vi "demoYouTubeCDSim.vi"() -> ()   [LabVIEW 2020]
uses:
  <vilib>/addons/Control Design/_Model Construction/Model Creation.llb/Model Creation SubVI/cd_Create Transfer Function Model.vi
  <vilib>/addons/Control Design/_Utility/Model Viewer.llb/Model Viewer SubVI/cd_Draw Transfer Function Equation (TF).vi
  <vilib>/addons/Control Design/_Model Construction/NI_LinSys_Model Creation.lvlib
  <vilib>/addons/Control Design/_Utility/NI_CD_Model Viewer.lvlib
panel:
  in  "Delay (custom)":dbl format="%#_13g"
  in  "Denominator Coeffs (custom)":dbl[](array[numeric])=[1.0, 4.0, 8.0, 7.0]
  in  "Numerator Coeffs (custom)":dbl[](array[numeric])=[10.0, 5.0]
  out "Transfer Function Eqn":picture
  in  "Which Transfer Function Do You Want?":T1(ring)
  in  "Stop Program":bool
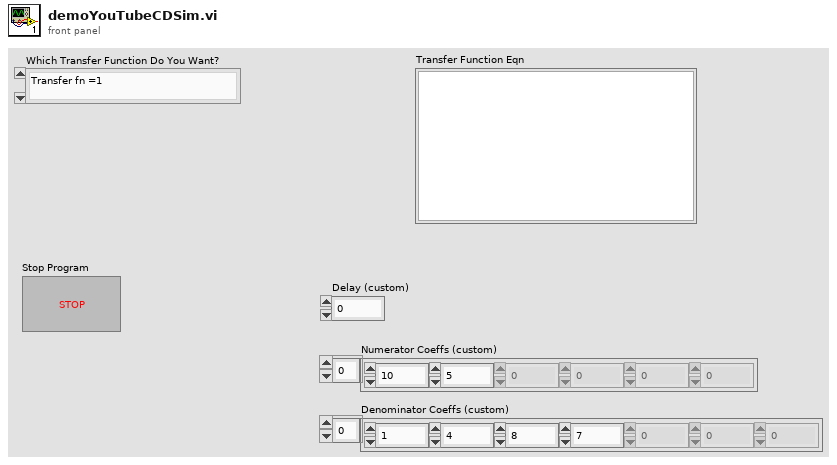
[diagram p1: front panel]
types:
  T1 = enum16{"Transfer fn =1", "first order with delay", "second order", "third order", "custom 1", "test 1", "test 2", "test 3", "test 4", "test 5", "test 6", "test 7", "test 8", "test 9", "test 10", ""}
  T2 = typedef "NI_LinSys_Model Typedefs.lvlib/CD Transfer Function Model (MIMO).ctl" = cluster{"properties":T3, "transfer function(s)":T4[][]}
  T3 = typedef "NI_LinSys_Model Typedefs.lvlib/CD General Elements.ctl" = cluster{"Model name":string, "Input names":string[], "Output names":string[], "Input Delays":dbl[], "Output Delays":dbl[], "Sampling Time":dbl, "Notes":string}
  T4 = typedef "NI_LinSys_Model Typedefs.lvlib/CD Transfer Function Model (SISO).ctl" = cluster{"Numerator":dbl[], "Denominator":dbl[], "delay":dbl}
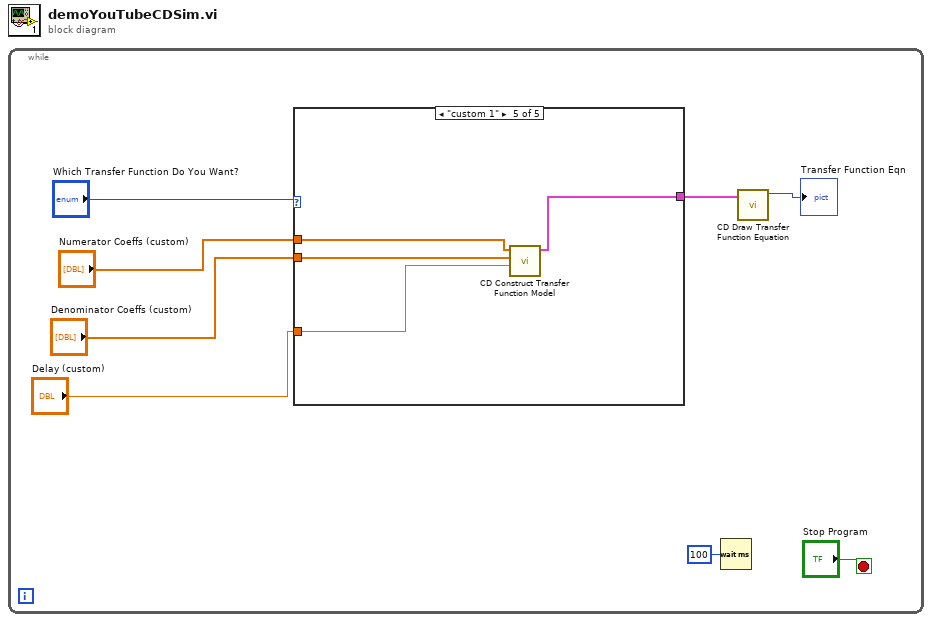
[diagram p0: block diagram]
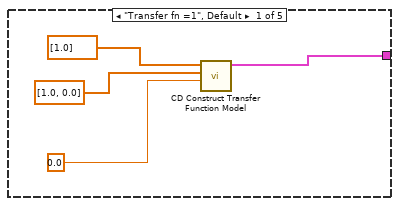
[diagram p2: hidden frame]
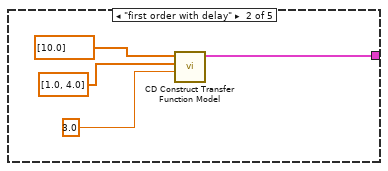
[diagram p3: hidden frame]
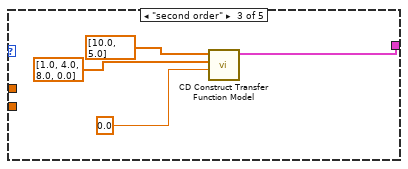
[diagram p4: hidden frame]
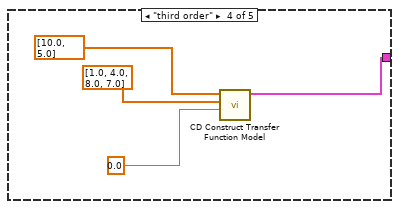
[diagram p5: hidden frame]
diagram:
  n1 = while {
    stop <- "Stop Program" stop-if-true
    n2 = case shown="\"custom 1\"" "Which Transfer Function Do You Want?" {
      tunnel: [w10 w13 w17 w21 w28] -> w4
      tunnel: "Numerator Coeffs (custom)" -> [_ _ _ _ w27]
      tunnel: "Denominator Coeffs (custom)" -> [_ _ _ _ w26]
      tunnel: "Delay (custom)" -> [_ _ _ _ w25]
      frame "Transfer fn =1", Default {
        n3 = call-poly <vilib>:"CD Construct Transfer Function Model.vi"("Delay"=0.0, "Denominator"=dbl[] [1.0, 0.0], "Numerator"=dbl[] [1.0]) -> ("Transfer Function Model"=w10:T2)  [unwired: 7 in, 1 out]
      }
      frame "first order with delay" {
        n4 = call-poly <vilib>:"CD Construct Transfer Function Model.vi"("Delay"=3.0, "Denominator"=dbl[] [1.0, 4.0], "Numerator"=dbl[] [10.0]) -> ("Transfer Function Model"=w13:T2)  [unwired: 7 in, 1 out]
      }
      frame "second order" {
        n5 = call-poly <vilib>:"CD Construct Transfer Function Model.vi"("Delay"=0.0, "Denominator"=dbl[] [1.0, 4.0, 8.0, 0.0], "Numerator"=dbl[] [10.0, 5.0]) -> ("Transfer Function Model"=w17:T2)  [unwired: 7 in, 1 out]
      }
      frame "third order" {
        n6 = call-poly <vilib>:"CD Construct Transfer Function Model.vi"("Delay"=0.0, "Denominator"=dbl[] [1.0, 4.0, 8.0, 7.0], "Numerator"=dbl[] [10.0, 5.0]) -> ("Transfer Function Model"=w21:T2)  [unwired: 7 in, 1 out]
      }
      frame "custom 1" {
        n7 = call-poly <vilib>:"CD Construct Transfer Function Model.vi"("Delay"=w25, "Denominator"=w26, "Numerator"=w27) -> ("Transfer Function Model"=w28:T2)  [unwired: 7 in, 1 out]
      }
    }
    n8 = Wait (ms)(milliseconds to wait=u32 100) -> ()  [unwired: 1 out]
    n9 = call-poly <vilib>:"CD Draw Transfer Function Equation.vi"("Transfer Function Model"=w4) -> ("Equation"=→"Transfer Function Eqn":picture)  [unwired: 8 in, 2 out]
  }
